vi "Initialize.vi"(7 "error in":errorcluster caption="错误输入（无错误）", 10 "PanelRootNode in":refnum<class "PanelRootNode.lvclass"> caption="LinkNode in") -> (0 "error out":errorcluster caption="错误输出", 2 "SelfNode*":refnum<data-value>)   [LabVIEW 2013, in "PanelRootNode.lvclass"]
uses:
  PanelRootNode.lvclass
  PanelLinkNode/PanelLinkNode.lvclass
  PanelDataNode/PanelDataNode.lvclass
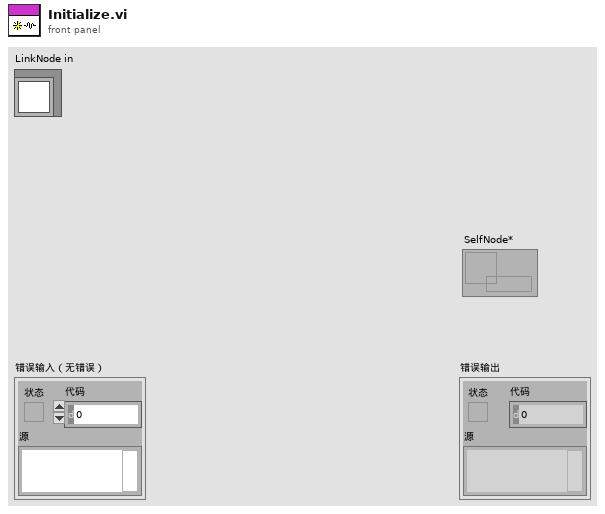
[diagram p1: front panel]
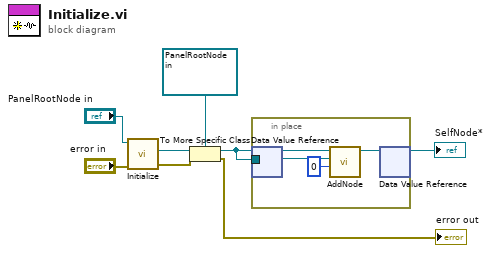
[diagram p0: block diagram]
diagram:
  n1 = call-parent "Initialize.vi"("error in"="error in", "PanelDataNode in"="PanelRootNode in") -> ("error out"=w5:errorcluster, "SelfNode*"=w6:refnum<data-value>)  [unwired: 7 in]
  n2 = To More Specific Class(target class=refnum<data-value> refnum ("数据值引用"), reference=w6, error in=w5) -> (specific class reference=w1:refnum<data-value>, error out=→"error out":errorcluster)
  n3 = in-place {
    in-place-border: w1 -> [w10]
    n4 = in-place-dvr #1(w1) -> (w12:refnum<class "PanelRootNode.lvclass">)  [unwired: 1 out]
    n5 = call "AddNode.vi"("Index"=0, "Node*"=w10, "PanelRootNode 输入"=w12) -> ("PanelRootNode 输出"=w11:refnum<class "PanelRootNode.lvclass">)  [unwired: 7 in, 1 out]
    n6 = in-place-dvr #1(w11) -> (→"SelfNode*":refnum<data-value>)  [unwired: 1 out]
  }
